vi "Normalize Input Polar.vi"(8 "V Input":dbl, 11 "U Input":dbl) -> (0 "Y Output":dbl, 3 "X Output":dbl)   [LabVIEW 2018]
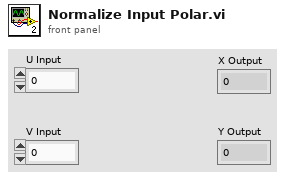
[diagram p1: front panel]
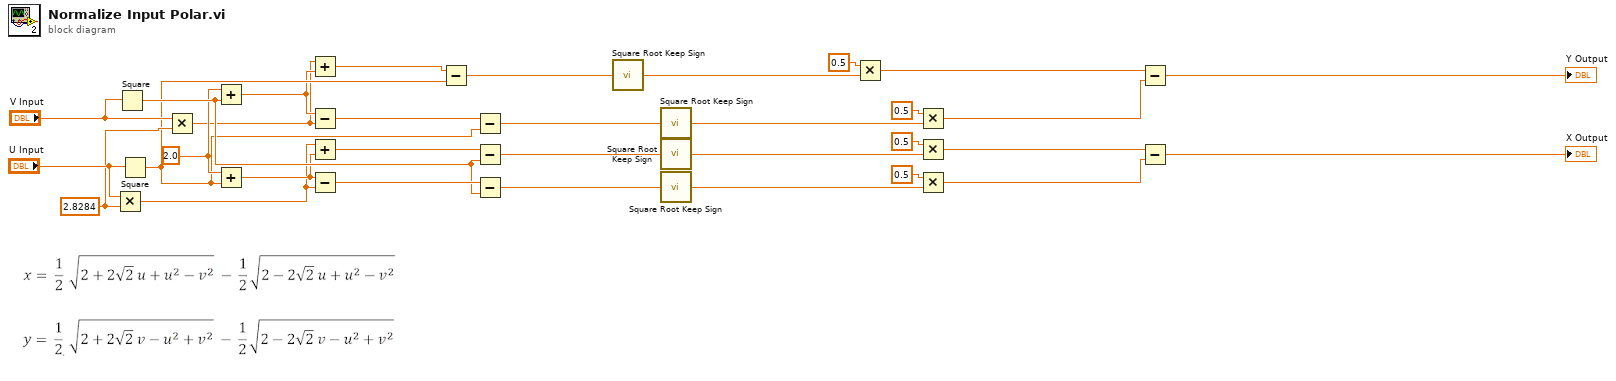
[diagram p0: block diagram]
diagram:
  w16 = 2.8284 ("value")
  w17 = 2.0 ("value")
  n1 = Multiply(x="U Input", y=w16) -> (x*y=w12:dbl)
  n2 = Square(x="V Input") -> (x^2=w18:dbl)
  n3 = Square(x="U Input") -> (x^2=w13:dbl)
  n4 = Multiply(x="V Input", y=w16) -> (x*y=w9:dbl)
  n5 = Add(x=w17, y=w18) -> (x+y=w11:dbl)
  n6 = Add(x=w17, y=w13) -> (x+y=w14:dbl)
  n7 = Add(x=w9, y=w11) -> (x+y=w10:dbl)
  n8 = Subtract(x=w11, y=w9) -> (x-y=w23:dbl)
  n9 = Add(x=w12, y=w14) -> (x+y=w15:dbl)
  n10 = Subtract(x=w14, y=w12) -> (x-y=w31:dbl)
  n11 = Subtract(x=w10, y=w13) -> (x-y=w3:dbl)
  n12 = Subtract(x=w23, y=w13) -> (x-y=w2:dbl)
  n13 = Subtract(x=w15, y=w18) -> (x-y=w8:dbl)
  n14 = Subtract(x=w31, y=w18) -> (x-y=w6:dbl)
  n15 = call "Square Root Keep Sign.vi"("Input"=w3) -> ("Square Root Save Sign"=w4:dbl)
  n16 = call "Square Root Keep Sign.vi"("Input"=w2) -> ("Square Root Save Sign"=w1:dbl)
  n17 = call "Square Root Keep Sign.vi"("Input"=w8) -> ("Square Root Save Sign"=w7:dbl)
  n18 = call "Square Root Keep Sign.vi"("Input"=w6) -> ("Square Root Save Sign"=w5:dbl)
  n19 = Multiply(x=0.5, y=w4) -> (x*y=w25:dbl)
  n20 = Multiply(x=0.5, y=w1) -> (x*y=w26:dbl)
  n21 = Multiply(x=0.5, y=w7) -> (x*y=w29:dbl)
  n22 = Multiply(x=0.5, y=w5) -> (x*y=w28:dbl)
  n23 = Subtract(x=w25, y=w26) -> (x-y=→"Y Output":dbl)
  n24 = Subtract(x=w29, y=w28) -> (x-y=→"X Output":dbl)
